vi "OCT Functinal Global.vi"(6 "Program Handle":T10, 7 "FFT States":T11, 8 "Error In":errorcluster, 9 "Input U16 Data":u16[][][](array[numeric]), 10 "Device In":T2, 11 "Dimension In":T4={"Depth"=1, "Height"=1000, "Width"=1024} {"Width" min=1; "Height" min=1; "Depth" min=1}) -> (0 "Error Out":errorcluster, 2 "Phase":sgl[][](array[numeric]), 3 "Magnitude":sgl[][](array[numeric]))   [LabVIEW 2012]
uses:
  User Controls/Array Dimensions.ctl
  Non-User VIs/Controls/Device ID.ctl
  OCT States.ctl
  Non-User VIs/Controls/Program Handle.ctl
  Non-User VIs/Controls/Memory Object.ctl
  Non-User VIs/Controls/Memory ID.ctl
  Non-User VIs/Controls/Memory Type.ctl
  Non-User VIs/FFT/FFT Control.ctl
  Non-User VIs/FFT/FFT Types.ctl
  Non-User VIs/FFT/FFT Dimension.ctl
  Non-User VIs/FFT/FFT Direction.ctl
  Non-User VIs/Allocate Memory/AllocateMemory_u16.vi
  Non-User VIs/Allocate Memory/AllocateMemory_32f.vi
  <vilib>/Analysis/4window.llb/Hanning Window (DBL).vi
  Non-User VIs/Write Memory/WriteMemory_32f.vi
  Non-User VIs/FFT/Create FFT Plan 32f.vi
  Non-User VIs/Write Memory/WriteMemory_u16.vi
  Non-User VIs/Set Kernel Arguments/Set Kernel Arguments Memory Object.vi
  Non-User VIs/Set Kernel Arguments/Set Kernel Arguments 32f.vi
  Non-User VIs/FFT/Compute FFT 32f.vi
  Non-User VIs/FFT/Delete FFT Plan 32f.vi
  Non-User VIs/Read Memory/ReadMemory_32f.vi
  OpenCLV x64.lvlib
  <vilib>/Analysis/NI_AALPro.lvlib
panel:
  out "Hanning Window":T1={"Device ID"=0, "Memeroy ID"=0, "Dimension"={"Depth"=1, "Height"=1, "Width"=1}, "Memory Type"=enum."32f"} {"Dimension"."Width" min=1; "Dimension"."Height" min=1; "Dimension"."Depth" min=1}
  out "FFT Object":T6 {"Imag"."Dimension"."Width" min=1; "Imag"."Dimension"."Height" min=1; "Imag"."Dimension"."Depth" min=1; "Real"."Dimension"."Width" min=1; "Real"."Dimension"."Height" min=1; "Real"."Dimension"."Depth" min=1}
  out "Program Handle 3":T10
  out "Pre FFT 32f":T1={"Device ID"=0, "Memeroy ID"=0, "Dimension"={"Depth"=1, "Height"=1, "Width"=1}, "Memory Type"=enum."32f"} {"Dimension"."Width" min=1; "Dimension"."Height" min=1; "Dimension"."Depth" min=1}
  out "u16 Input":T1={"Device ID"=0, "Memeroy ID"=0, "Dimension"={"Depth"=1, "Height"=1, "Width"=1}, "Memory Type"=enum."32f"} {"Dimension"."Width" min=1; "Dimension"."Height" min=1; "Dimension"."Depth" min=1}
  in  "Imag":T1={"Device ID"=0, "Memeroy ID"=0, "Dimension"={"Depth"=1, "Height"=1, "Width"=1}, "Memory Type"=enum."32f"} {"Dimension"."Width" min=1; "Dimension"."Height" min=1; "Dimension"."Depth" min=1}
  in  "Real":T1={"Device ID"=0, "Memeroy ID"=0, "Dimension"={"Depth"=1, "Height"=1, "Width"=1}, "Memory Type"=enum."32f"} {"Dimension"."Width" min=1; "Dimension"."Height" min=1; "Dimension"."Depth" min=1}
  out "Program Handle 2":T10
  # "Locals"
  # "Outputs"
  # "Inputs"
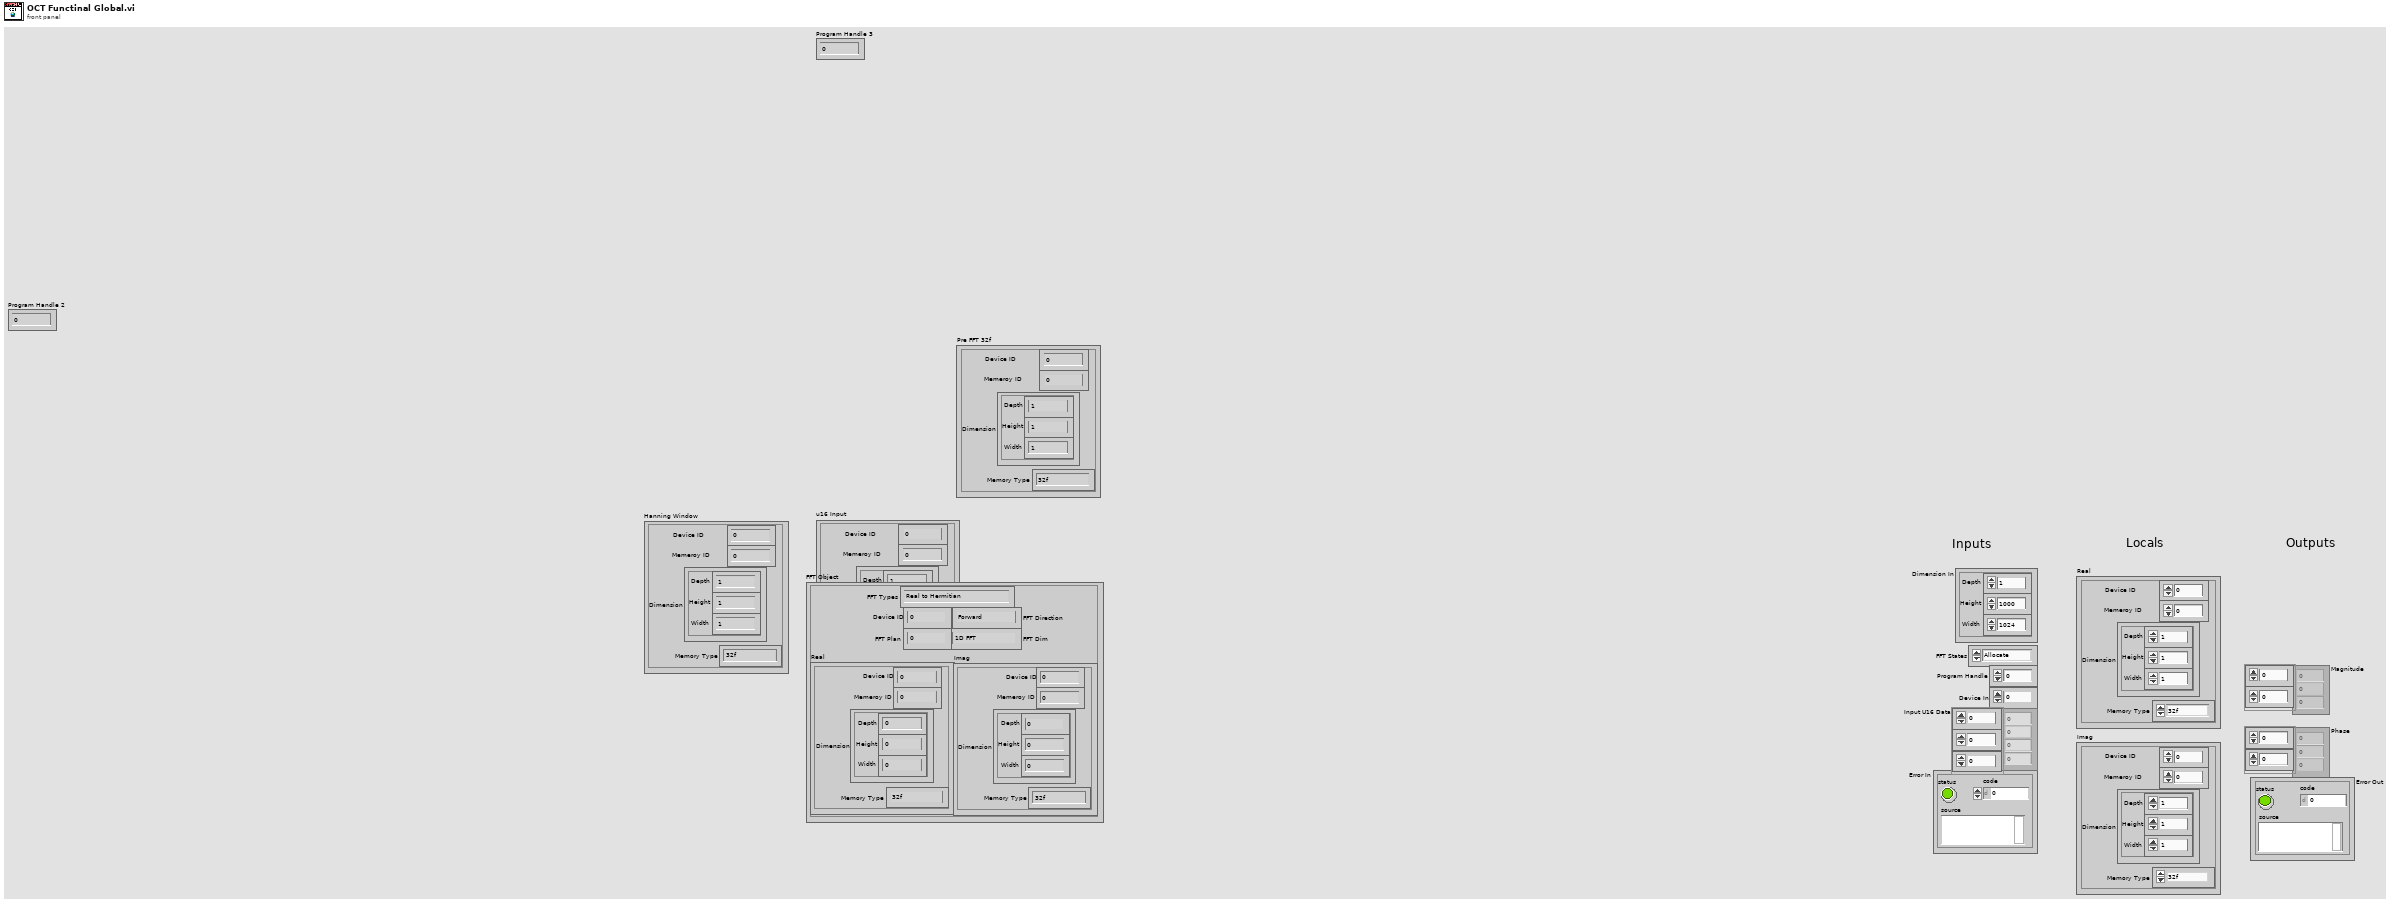
[diagram p1: front panel]
types:
  T1 = typedef "OpenCLV x64.lvlib/Memory Object.ctl" = cluster{"Device ID":T2, "Memeroy ID":T3, "Dimension":T4, "Memory Type":T5}
  T2 = typedef "OpenCLV x64.lvlib/Device ID.ctl" = u64
  T3 = typedef "OpenCLV x64.lvlib/Memory ID.ctl" = u64
  T4 = typedef "Array Dimensions.ctl" = cluster{"Depth":u64, "Height":u64, "Width":u64}
  T5 = typedef "OpenCLV x64.lvlib/Memory Type.ctl" = enum16{"32f", "u8", "i8", "u16", "i16", "u32", "i32", "64f"}
  T6 = typedef "OpenCLV x64.lvlib/FFT Control.ctl" = cluster{"Device ID":T2, "FFT Types":T7, "FFT Dim":T8, "Real":T1, "Imag":T1, "FFT Plan":u64, "FFT Direction":T9}
  T7 = typedef "OpenCLV x64.lvlib/FFT Types.ctl" = enum16{"Real to Hermitian", "Hermitian to Real", "Complex to Complex"}
  T8 = typedef "OpenCLV x64.lvlib/FFT Dimension.ctl" = enum16{"1D FFT", "2D FFT", "3D FFT"}
  T9 = typedef "OpenCLV x64.lvlib/FFT Direction.ctl" = enum16{"Forward", "Reverse"}
  T10 = typedef "OpenCLV x64.lvlib/Program Handle.ctl" = u64
  T11 = typedef "OCT States.ctl" = enum16{"Allocate", "Pre-FFT No Optimization", "Pre-FFT Global Memory", "Pre-FFT Local Memory", "FFT", "Post FFT", "Read Data", "Clean-up"}
  T12 = cluster{"Memory Object":T1, "Memory Object":T1, "Memory Object Out":T1, "FFT Object":T6, "Memory Object":T1, "Memory Object":T1, "Real":T1, "Imag":T1}
  T13 = typedef "OpenCLV x64.lvlib/Kernel Handle.ctl" = u64
  T14 = typedef "OpenCLV x64.lvlib/Kernel Workgroup Information.ctl" = cluster{"Compile Workgroup Size":u64[], "Kernel Private Mem":u64, "Kernel Local Mem":u64, "Work Group Multiple":u64, "Max Work Group Size":u64}
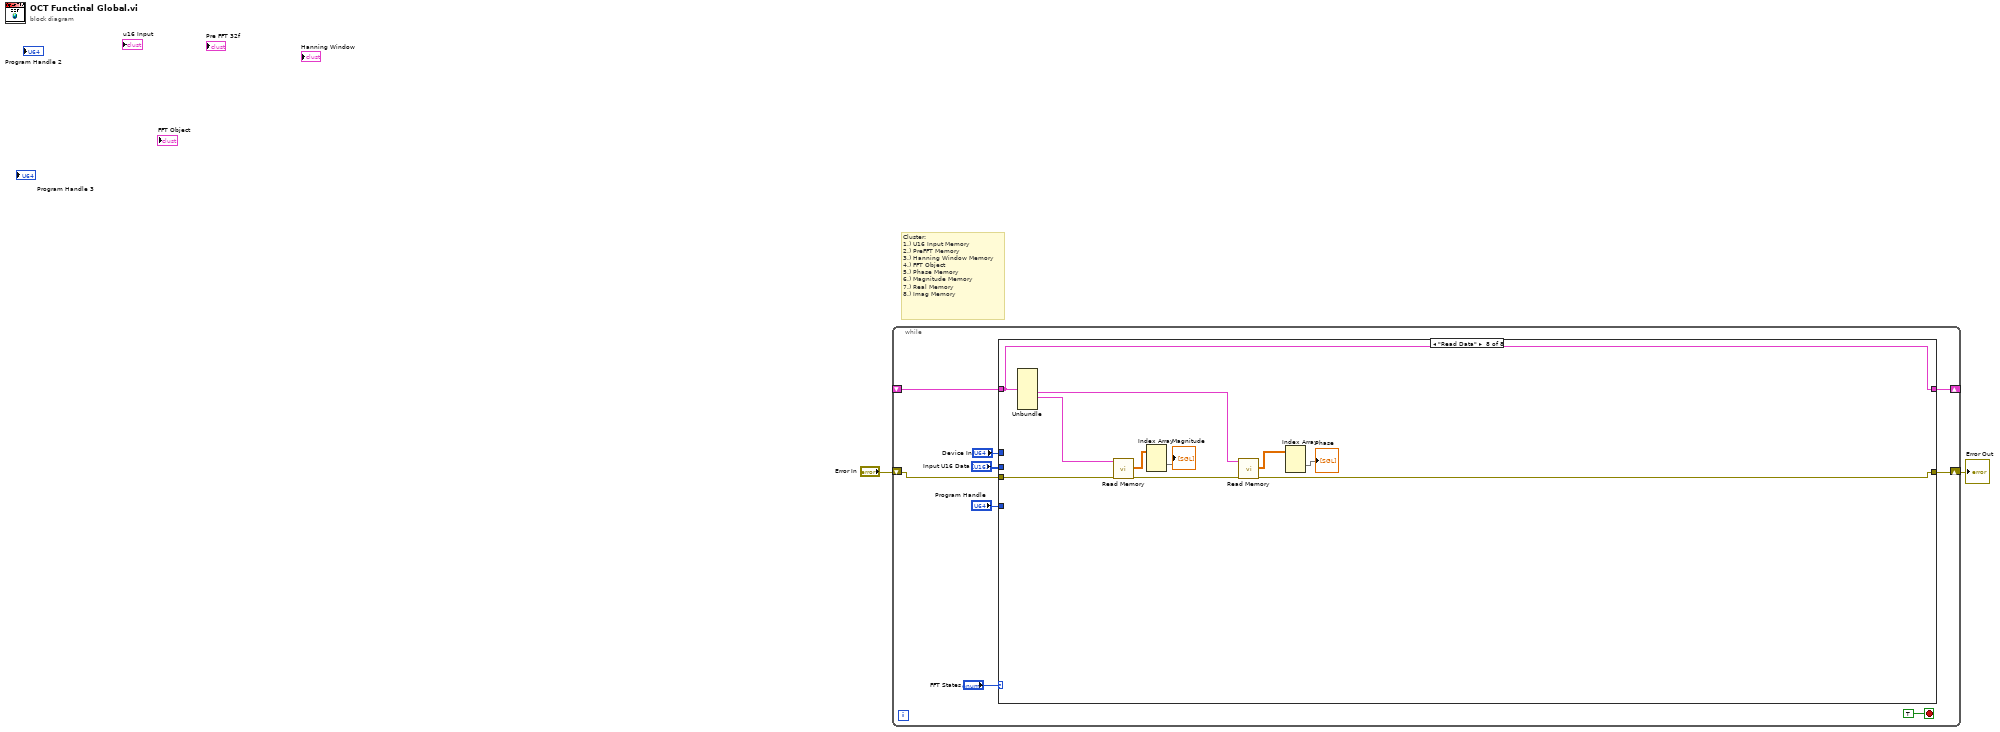
[diagram p0: block diagram]
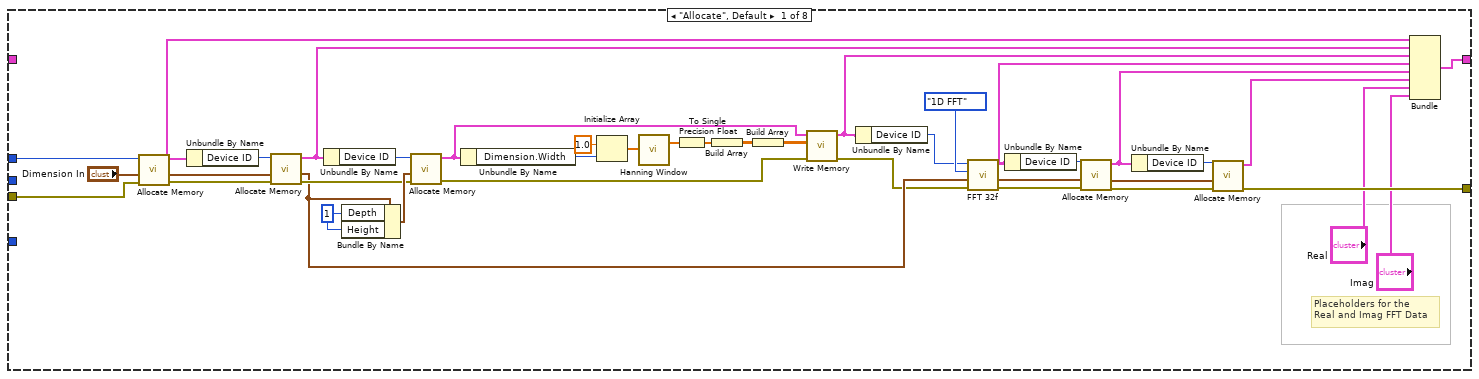
[diagram p2: hidden frame]
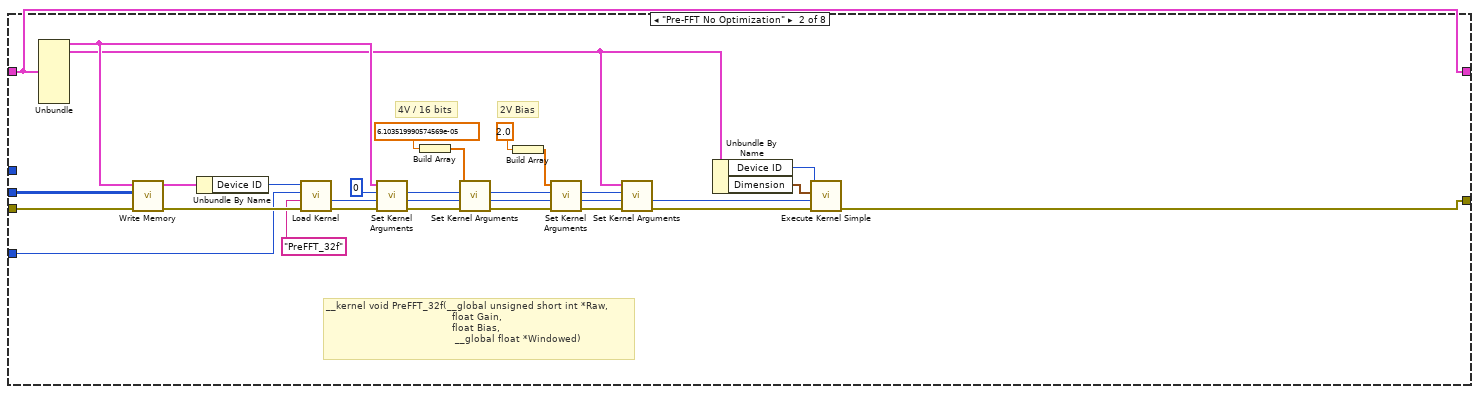
[diagram p3: hidden frame]
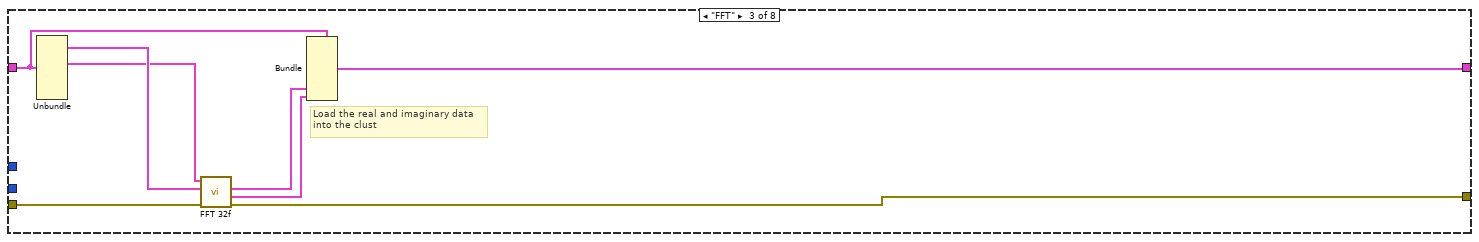
[diagram p4: hidden frame]
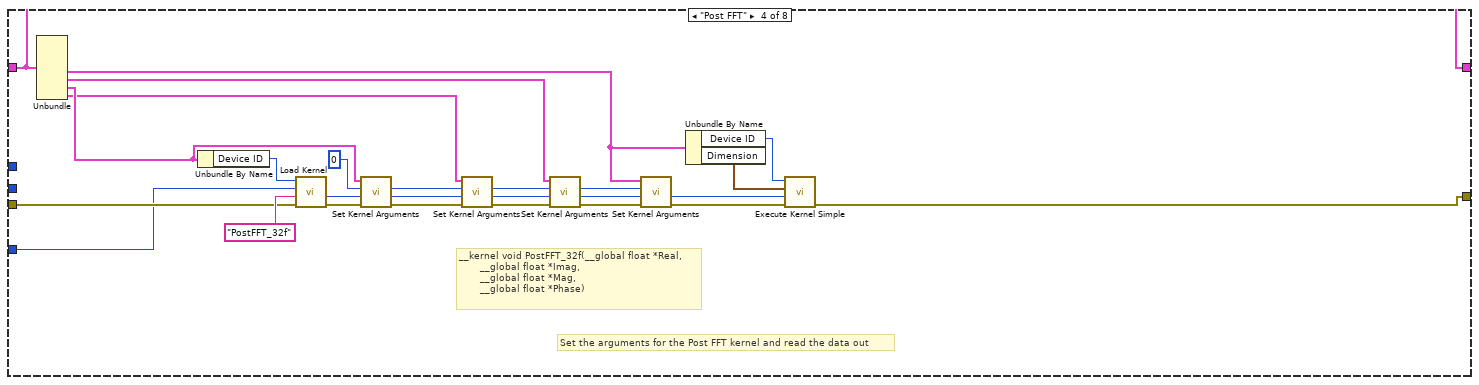
[diagram p5: hidden frame]
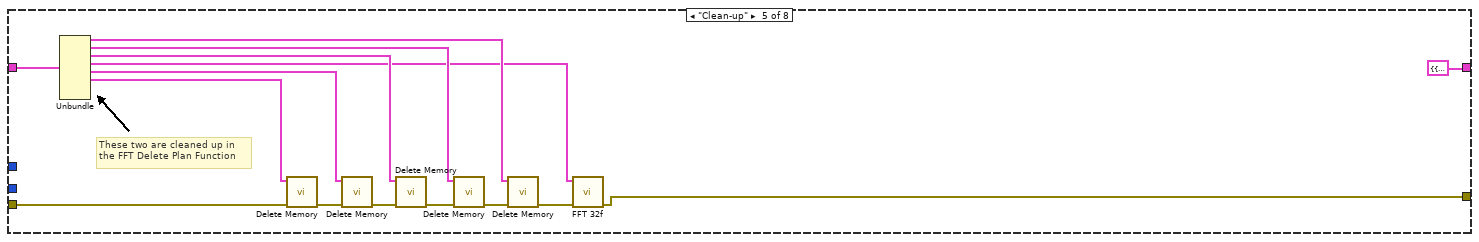
[diagram p6: hidden frame]
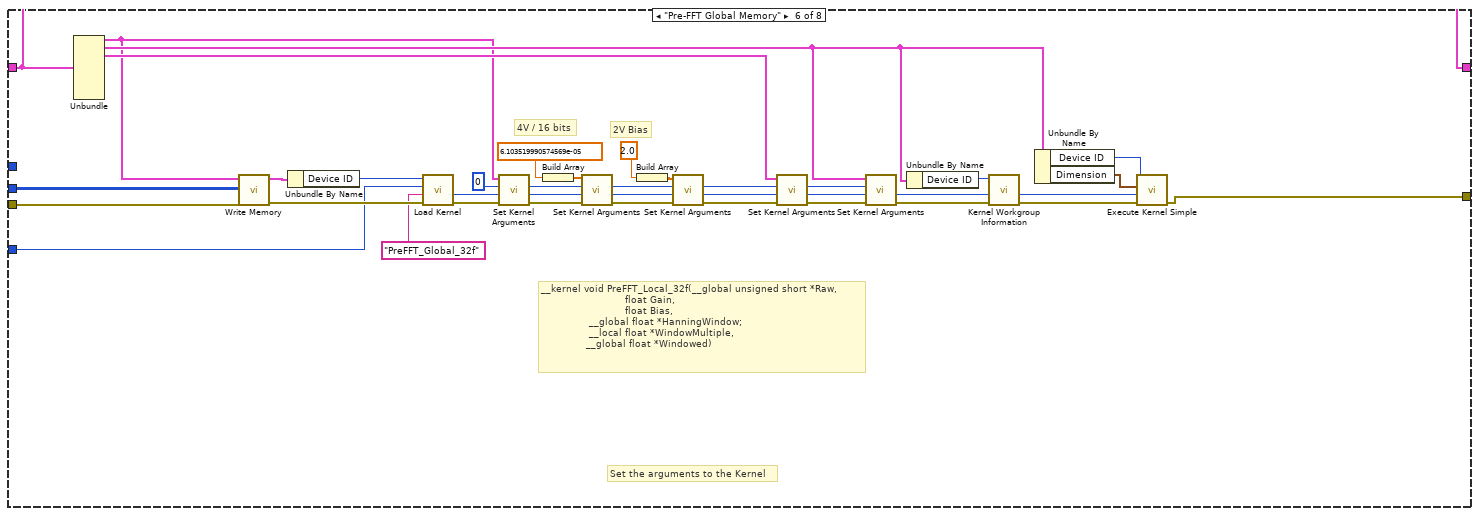
[diagram p7: hidden frame]
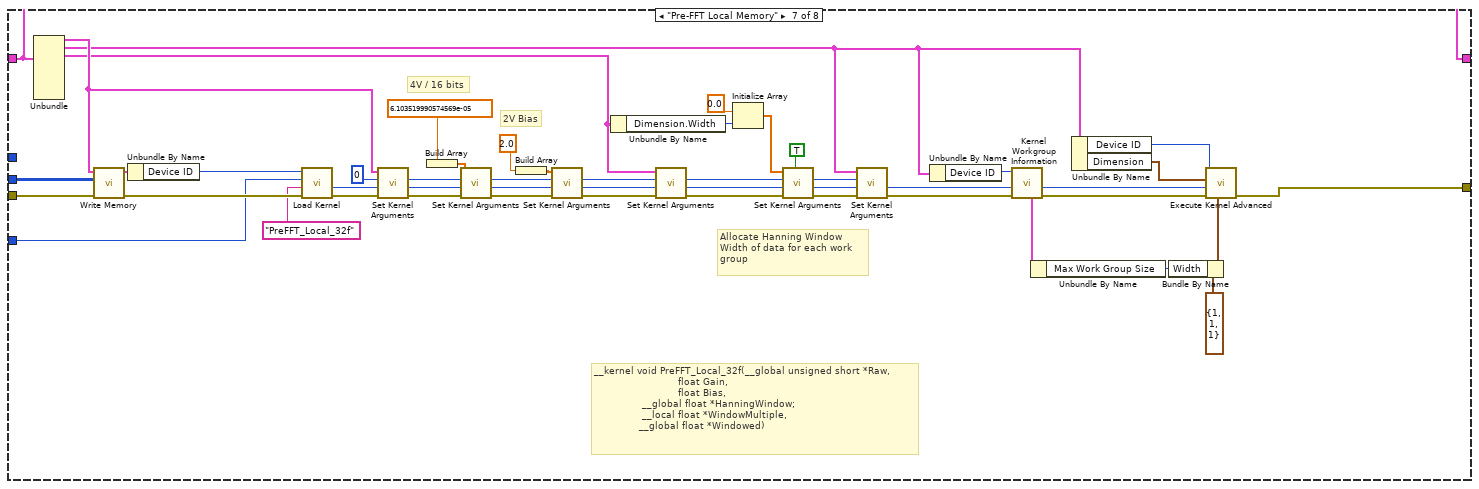
[diagram p8: hidden frame]
diagram:
  # "Cluster:\n1.) U16 Input Memory\n2.) PreFFT Memory\n3.) Hanning Window Memory\n4.) FFT Object\n5.) Phase Memory\n6.) Magnitude Memory\n7.) Real Memory\n8.) Imag Memory"
  n1 = while {
    shift-right: [w8] -> _
    shift-left: _ -> [w7]
    shift-right: [w6] -> w1
    shift-left: "Error In" -> [w5]
    stop <- TRUE stop-if-true
    n2 = case shown="\"Read Data\"" "FFT States" {
      tunnel: "Device In" -> [w27 _ _ _ _ _ _ _]
      tunnel: [w16 w56 w82 w92 T12 {"Memory Object"={"Device ID"=0, "Memeroy ID"=0, "Dimension"={"Depth"=0, "Height"=0, "Width"=0}, "Memory Type"=enum."32f"}, "Memory Object"={"Device ID"=0, "Memeroy ID"=0, "Dimension"={"Depth"=0, "Height"=0, "Width"=0}, "Memory Type"=enum."32f"}, "Memory Object Out"={"Device ID"=0, "Memeroy ID"=0, "Dimension"={"Depth"=0, "Height"=0, "Width"=0}, "Memory Type"=enum."32f"}, "FFT Object"={"Device ID"=0, "FFT Types"=enum."Real to Hermitian", "FFT Dim"=enum."1D FFT", "Real"={"Device ID"=0, "Memeroy ID"=0, "Dimension"={"Depth"=0, "Height"=0, "Width"=0}, "Memory Type"=enum."32f"}, "Imag"={"Device ID"=0, "Memeroy ID"=0, "Dimension"={"Depth"=0, "Height"=0, "Width"=0}, "Memory Type"=enum."32f"}, "FFT Plan"=0, "FFT Direction"=enum."Forward"}, "Memory Object"={"Device ID"=0, "Memeroy ID"=0, "Dimension"={"Depth"=0, "Height"=0, "Width"=0}, "Memory Type"=enum."32f"}, "Memory Object"={"Device ID"=0, "Memeroy ID"=0, "Dimension"={"Depth"=0, "Height"=0, "Width"=0}, "Memory Type"=enum."32f"}, "Real"={"Device ID"=0, "Memeroy ID"=0, "Dimension"={"Depth"=0, "Height"=0, "Width"=0}, "Memory Type"=enum."32f"}, "Imag"={"Device ID"=0, "Memeroy ID"=0, "Dimension"={"Depth"=0, "Height"=0, "Width"=0}, "Memory Type"=enum."32f"}} ("Cluster") w133 w217 w218] -> w8
      tunnel: w7 -> [_ w56 w85 w92 w129 w133 w217 w218]
      tunnel: w5 -> [w15 w58 w89 w97 w116 w139 w177 w225]
      tunnel: [w14 w55 w86 w91 w117 w134 w171 w222] -> w6
      tunnel: "Program Handle" -> [_ w57 _ w90 _ w135 w175 _]
      tunnel: "Input U16 Data" -> [_ w52 _ _ _ w131 w176 _]
      frame "Allocate", Default {
        w42 = u64 1 ("Depth")
        # "Placeholders for the \nReal and Imag FFT Data"
        n3 = call-poly "Allocate Memory.vi"("Error In"=w15, "Dimension"="Dimension In", "Device In"=w27) -> ("Error Out"=w35:errorcluster, "Dimension Out"=w36:T4, "Memory Object"=w24:T1)  [unwired: 6 in]
        n4 = Unbundle By Name(w24) -> ("Device ID"=w34:T2)
        n5 = call-poly "Allocate Memory.vi"("Error In"=w35, "Dimension"=w36, "Device In"=w34) -> ("Error Out"=w39:errorcluster, "Dimension Out"=w23:T4, "Memory Object"=w26:T1)  [unwired: 6 in]
        n6 = Unbundle By Name(w26) -> ("Device ID"=w43:T2)
        n7 = Bundle By Name(cluster=w23, "Depth"=w42, "Height"=w42) -> (w40:T4)
        n8 = call-poly "Allocate Memory.vi"("Error In"=w39, "Dimension"=w40, "Device In"=w43) -> ("Error Out"=w28:errorcluster, "Memory Object"=w25:T1)  [unwired: 6 in, 1 out]
        n9 = Unbundle By Name(w25) -> ("Dimension.Width"=w48:u64)
        n10 = Initialize Array(1.0 ("element"), w48) -> (w49:dbl[])
        n11 = call-poly <vilib>:"Hanning Window.vi"("X"=w49) -> ("Windowed X"=w46:dbl[])  [unwired: 1 out]
        n12 = To Single Precision Float(number=w46) -> (single precision float=w45:sgl[])
        n13 = Build Array(w45) -> (w44:sgl[][])
        n14 = Build Array(w44) -> (w50:sgl[][][])
        n15 = call-poly "Write Memory.vi"("Error In"=w28, "Data In"=w50, "Memory Object In"=w25) -> ("Error Out"=w22:errorcluster, "Memory Object Out"=w21:T1)  [unwired: 6 in, 1 out]
        n16 = Unbundle By Name(w21) -> ("Device ID"=w20:T2)
        n17 = call-poly "FFT 32f.vi"("Error In"=w22, "Dimension"=w23, "FFT Dimension"=FFT_Dimension."1D FFT", "Labview Device"=w20) -> ("Error Out"=w30:errorcluster, "FFT Output Dimensions"=w37:T4, "FFT Object"=w19:T6)  [unwired: 5 in]
        n18 = Unbundle By Name(w19) -> ("Device ID"=w38:T2)
        n19 = call-poly "Allocate Memory.vi"("Error In"=w30, "Dimension"=w37, "Device In"=w38) -> ("Error Out"=w33:errorcluster, "Dimension Out"=w32:T4, "Memory Object"=w18:T1)  [unwired: 6 in]
        n20 = Unbundle By Name(w18) -> ("Device ID"=w31:T2)
        n21 = call-poly "Allocate Memory.vi"("Error In"=w33, "Dimension"=w32, "Device In"=w31) -> ("Error Out"=w14:errorcluster, "Memory Object"=w17:T1)  [unwired: 6 in, 1 out]
        n22 = Bundle("Memory Object"=w24, "Memory Object"=w26, "Memory Object Out"=w21, "FFT Object"=w19, "Memory Object"=w18, "Memory Object"=w17, "Real"="Real", "Imag"="Imag") -> (w16:T12)  [unwired: 1 in]
      }
      frame "Pre-FFT No Optimization" {
        # "2V Bias"
        # "4V / 16 bits"
        # "__kernel void PreFFT_32f(__global unsigned short int *Raw,\n                                          float Gain,\n                                          float Bias,\n\t\t\t                                        __global float *Windowed)"
        n23 = Unbundle(w56) -> ("Memory Object"=w53:T1, "Memory Object"=w51:T1)  [unwired: 6 out]
        n24 = call-poly "Write Memory.vi"("Error In"=w58, "Data In"=w52, "Memory Object In"=w53) -> ("Error Out"=w69:errorcluster, "Memory Object Out"=w54:T1)  [unwired: 7 in]
        n25 = Unbundle By Name(w54) -> ("Device ID"=w78:T2)
        n26 = call "Load Kernel.vi"("Error In"=w69, "Kernel Name"="PreFFT_32f", "Program Handle"=w57, "Device In"=w78) -> ("Error Out"=w81:errorcluster, "Kernel Handle"=w80:T13)  [unwired: 4 in, 2 out]
        n27 = call-poly "Set Kernel Arguments.vi"("Error In"=w81, "Kernel Handle"=w80, "Argument Number"=0, "Memory Object"=w53) -> ("Error Out"=w60:errorcluster, "Kernel Handle out"=w72:T13, "Auto Inc Arugment Number"=w73:i32)  [unwired: 5 in]
        n28 = Build Array(sgl 6.10352e-05 ("x")) -> (w61:sgl[])
        n29 = call-poly "Set Kernel Arguments.vi"("Error In"=w60, "Kernel Handle"=w72, "Argument Number"=w73, "32f Constant"=w61) -> ("Error Out"=w63:errorcluster, "Kernel Handle out"=w71:T13, "Auto Inc Arugment Number"=w74:i32)  [unwired: 5 in]
        n30 = Build Array(sgl 2.0 ("x")) -> (w62:sgl[])
        n31 = call-poly "Set Kernel Arguments.vi"("Error In"=w63, "Kernel Handle"=w71, "Argument Number"=w74, "32f Constant"=w62) -> ("Error Out"=w64:errorcluster, "Kernel Handle out"=w65:T13, "Auto Inc Arugment Number"=w66:i32)  [unwired: 5 in]
        n32 = call-poly "Set Kernel Arguments.vi"("Error In"=w64, "Kernel Handle"=w65, "Argument Number"=w66, "Memory Object"=w51) -> ("Error Out"=w67:errorcluster, "Kernel Handle out"=w77:T13)  [unwired: 5 in, 1 out]
        n33 = Unbundle By Name(w51) -> ("Device ID"=w68:T2, "Dimension"=w70:T4)
        n34 = call "Execute Kernel Simple.vi"("Error In"=w67, "Kernel Handle"=w77, "Thread Dimensions"=w70, "Device In"=w68) -> ("Error Out"=w55:errorcluster)  [unwired: 4 in, 3 out]
      }
      frame "FFT" {
        # "Load the real and imaginary data\ninto the clust"
        n35 = Unbundle(w85) -> ("Memory Object"=w88:T1, "FFT Object"=w87:T6)  [unwired: 6 out]
        n36 = call-poly "FFT 32f.vi"("Error In"=w89, "Real In"=w88, "FFT Object"=w87) -> ("Error Out"=w86:errorcluster, "Imag Out"=w84:T1, "Real Out"=w83:T1)  [unwired: 4 in, 2 out]
        n37 = Bundle(cluster=w85, "Real"=w83, "Imag"=w84) -> (w82:T12)  [unwired: 6 in]
      }
      frame "Post FFT" {
        # "Set the arguments for the Post FFT kernel and read the data out"
        # "__kernel void PostFFT_32f(__global float *Real,\n\t\t\t    __global float *Imag,\n\t\t\t    __global float *Mag,\n    \t\t\t__global float *Phase)"
        n38 = Unbundle(w92) -> ("Memory Object"=w93:T1, "Memory Object"=w94:T1, "Real"=w96:T1, "Imag"=w95:T1)  [unwired: 4 out]
        n39 = Unbundle By Name(w96) -> ("Device ID"=w115:T2)
        n40 = call "Load Kernel.vi"("Error In"=w97, "Kernel Name"="PostFFT_32f", "Program Handle"=w90, "Device In"=w115) -> ("Error Out"=w99:errorcluster, "Kernel Handle"=w112:T13)  [unwired: 4 in, 2 out]
        n41 = call-poly "Set Kernel Arguments.vi"("Error In"=w99, "Kernel Handle"=w112, "Argument Number"=0, "Memory Object"=w96) -> ("Error Out"=w102:errorcluster, "Kernel Handle out"=w101:T13, "Auto Inc Arugment Number"=w100:i32)  [unwired: 5 in]
        n42 = call-poly "Set Kernel Arguments.vi"("Error In"=w102, "Kernel Handle"=w101, "Argument Number"=w100, "Memory Object"=w95) -> ("Error Out"=w103:errorcluster, "Kernel Handle out"=w104:T13, "Auto Inc Arugment Number"=w105:i32)  [unwired: 5 in]
        n43 = call-poly "Set Kernel Arguments.vi"("Error In"=w103, "Kernel Handle"=w104, "Argument Number"=w105, "Memory Object"=w94) -> ("Error Out"=w106:errorcluster, "Kernel Handle out"=w107:T13, "Auto Inc Arugment Number"=w108:i32)  [unwired: 5 in]
        n44 = call-poly "Set Kernel Arguments.vi"("Error In"=w106, "Kernel Handle"=w107, "Argument Number"=w108, "Memory Object"=w93) -> ("Error Out"=w109:errorcluster, "Kernel Handle out"=w114:T13)  [unwired: 5 in, 1 out]
        n45 = Unbundle By Name(w93) -> ("Device ID"=w110:T2, "Dimension"=w113:T4)
        n46 = call "Execute Kernel Simple.vi"("Error In"=w109, "Kernel Handle"=w114, "Thread Dimensions"=w113, "Device In"=w110) -> ("Error Out"=w91:errorcluster)  [unwired: 4 in, 3 out]
      }
      frame "Clean-up" {
        # "These two are cleaned up in\nthe FFT Delete Plan Function"
        n47 = Unbundle(w129) -> ("Memory Object"=w120:T1, "Memory Object"=w122:T1, "Memory Object Out"=w124:T1, "FFT Object"=w118:T6, "Memory Object"=w126:T1, "Memory Object"=w128:T1)  [unwired: 2 out]
        n48 = call "Delete Memory.vi"("Error In"=w116, "Memory Object In"=w128) -> ("Error Out"=w127:errorcluster)  [unwired: 8 in, 1 out]
        n49 = call "Delete Memory.vi"("Error In"=w127, "Memory Object In"=w126) -> ("Error Out"=w125:errorcluster)  [unwired: 8 in, 1 out]
        n50 = call "Delete Memory.vi"("Error In"=w125, "Memory Object In"=w124) -> ("Error Out"=w123:errorcluster)  [unwired: 8 in, 1 out]
        n51 = call "Delete Memory.vi"("Error In"=w123, "Memory Object In"=w122) -> ("Error Out"=w121:errorcluster)  [unwired: 8 in, 1 out]
        n52 = call "Delete Memory.vi"("Error In"=w121, "Memory Object In"=w120) -> ("Error Out"=w119:errorcluster)  [unwired: 8 in, 1 out]
        n53 = call-poly "FFT 32f.vi"("Error In"=w119, "FFT Object"=w118) -> ("Error Out"=w117:errorcluster)  [unwired: 9 in]
      }
      frame "Pre-FFT Global Memory" {
        # "2V Bias"
        # "4V / 16 bits"
        # "Set the arguments to the Kernel"
        # "__kernel void PreFFT_Local_32f(__global unsigned short *Raw,\n                           \tfloat Gain,\n                           \tfloat Bias,\n\t\t\t\t\t\t\t         __global float *HanningWindow;\n\t\t\t\t            __local float *WindowMultiple,\n\t\t           \t __global float *Windowed)"
        n54 = Unbundle(w133) -> ("Memory Object"=w132:T1, "Memory Object"=w137:T1, "Memory Object Out"=w138:T1)  [unwired: 5 out]
        n55 = call-poly "Write Memory.vi"("Error In"=w139, "Data In"=w131, "Memory Object In"=w132) -> ("Error Out"=w164:errorcluster, "Memory Object Out"=w136:T1)  [unwired: 7 in]
        n56 = Unbundle By Name(w136) -> ("Device ID"=w152:T2)
        n57 = call "Load Kernel.vi"("Error In"=w164, "Kernel Name"="PreFFT_Global_32f", "Program Handle"=w135, "Device In"=w152) -> ("Error Out"=w155:errorcluster, "Kernel Handle"=w154:T13)  [unwired: 4 in, 2 out]
        n58 = call-poly "Set Kernel Arguments.vi"("Error In"=w155, "Kernel Handle"=w154, "Argument Number"=0, "Memory Object"=w132) -> ("Error Out"=w141:errorcluster, "Kernel Handle out"=w147:T13, "Auto Inc Arugment Number"=w148:i32)  [unwired: 5 in]
        n59 = Build Array(sgl 6.10352e-05 ("x")) -> (w142:sgl[])
        n60 = call-poly "Set Kernel Arguments.vi"("Error In"=w141, "Kernel Handle"=w147, "Argument Number"=w148, "32f Constant"=w142) -> ("Error Out"=w144:errorcluster, "Kernel Handle out"=w146:T13, "Auto Inc Arugment Number"=w149:i32)  [unwired: 5 in]
        n61 = Build Array(sgl 2.0 ("x")) -> (w143:sgl[])
        n62 = call-poly "Set Kernel Arguments.vi"("Error In"=w144, "Kernel Handle"=w146, "Argument Number"=w149, "32f Constant"=w143) -> ("Error Out"=w161:errorcluster, "Kernel Handle out"=w162:T13, "Auto Inc Arugment Number"=w163:i32)  [unwired: 5 in]
        n63 = call-poly "Set Kernel Arguments.vi"("Error In"=w161, "Kernel Handle"=w162, "Argument Number"=w163, "Memory Object"=w138) -> ("Error Out"=w166:errorcluster, "Kernel Handle out"=w167:T13, "Auto Inc Arugment Number"=w168:i32)  [unwired: 5 in]
        n64 = call-poly "Set Kernel Arguments.vi"("Error In"=w166, "Kernel Handle"=w167, "Argument Number"=w168, "Memory Object"=w137) -> ("Error Out"=w156:errorcluster, "Kernel Handle out"=w157:T13)  [unwired: 5 in, 1 out]
        n65 = Unbundle By Name(w137) -> ("Device ID"=w160:T2)
        n66 = call "Kernel Workgroup Information.vi"("Error In"=w156, "Kernel Handle"=w157, "Device ID"=w160) -> ("Error Out"=w158:errorcluster, "Kernel Handle"=w159:T13)  [unwired: 5 in, 2 out]
        n67 = Unbundle By Name(w137) -> ("Device ID"=w145:T2, "Dimension"=w165:T4)
        n68 = call "Execute Kernel Simple.vi"("Error In"=w158, "Kernel Handle"=w159, "Thread Dimensions"=w165, "Device In"=w145) -> ("Error Out"=w134:errorcluster)  [unwired: 4 in, 3 out]
      }
      frame "Pre-FFT Local Memory" {
        # "Allocate Hanning Window\nWidth of data for each work\ngroup"
        # "2V Bias"
        # "4V / 16 bits"
        # "__kernel void PreFFT_Local_32f(__global unsigned short *Raw,\n                           \tfloat Gain,\n                           \tfloat Bias,\n\t\t\t\t\t\t\t         __global float *HanningWindow;\n\t\t\t\t            __local float *WindowMultiple,\n\t\t           \t __global float *Windowed)"
        n69 = Unbundle(w217) -> ("Memory Object"=w173:T1, "Memory Object"=w172:T1, "Memory Object Out"=w170:T1)  [unwired: 5 out]
        n70 = call-poly "Write Memory.vi"("Error In"=w177, "Data In"=w176, "Memory Object In"=w173) -> ("Error Out"=w190:errorcluster, "Memory Object Out"=w174:T1)  [unwired: 7 in]
        n71 = Unbundle By Name(w174) -> ("Device ID"=w180:T2)
        n72 = call "Load Kernel.vi"("Error In"=w190, "Kernel Name"="PreFFT_Local_32f", "Program Handle"=w175, "Device In"=w180) -> ("Error Out"=w182:errorcluster, "Kernel Handle"=w181:T13)  [unwired: 4 in, 2 out]
        n73 = call-poly "Set Kernel Arguments.vi"("Error In"=w182, "Kernel Handle"=w181, "Argument Number"=0, "Memory Object"=w173) -> ("Error Out"=w194:errorcluster, "Kernel Handle out"=w199:T13, "Auto Inc Arugment Number"=w200:i32)  [unwired: 5 in]
        n74 = Build Array(sgl 6.10352e-05 ("x")) -> (w195:sgl[])
        n75 = call-poly "Set Kernel Arguments.vi"("Error In"=w194, "Kernel Handle"=w199, "Argument Number"=w200, "32f Constant"=w195) -> ("Error Out"=w197:errorcluster, "Kernel Handle out"=w198:T13, "Auto Inc Arugment Number"=w201:i32)  [unwired: 5 in]
        n76 = Build Array(sgl 2.0 ("x")) -> (w196:sgl[])
        n77 = call-poly "Set Kernel Arguments.vi"("Error In"=w197, "Kernel Handle"=w198, "Argument Number"=w201, "32f Constant"=w196) -> ("Error Out"=w209:errorcluster, "Kernel Handle out"=w210:T13, "Auto Inc Arugment Number"=w211:i32)  [unwired: 5 in]
        n78 = Unbundle By Name(w170) -> ("Dimension.Width"=w169:u64)
        n79 = call-poly "Set Kernel Arguments.vi"("Error In"=w209, "Kernel Handle"=w210, "Argument Number"=w211, "Memory Object"=w170) -> ("Error Out"=w212:errorcluster, "Kernel Handle out"=w213:T13, "Auto Inc Arugment Number"=w214:i32)  [unwired: 5 in]
        n80 = Initialize Array(sgl 0.0 ("element"), w169) -> (w216:sgl[])
        n81 = call-poly "Set Kernel Arguments.vi"("Local Data?"=TRUE, "Error In"=w212, "Kernel Handle"=w213, "Argument Number"=w214, "32f Constant"=w216) -> ("Error Out"=w206:errorcluster, "Kernel Handle out"=w207:T13, "Auto Inc Arugment Number"=w208:i32)  [unwired: 4 in]
        n82 = call-poly "Set Kernel Arguments.vi"("Error In"=w206, "Kernel Handle"=w207, "Argument Number"=w208, "Memory Object"=w172) -> ("Error Out"=w183:errorcluster, "Kernel Handle out"=w184:T13)  [unwired: 5 in, 1 out]
        n83 = Unbundle By Name(w172) -> ("Device ID"=w187:T2)
        n84 = call "Kernel Workgroup Information.vi"("Error In"=w183, "Kernel Handle"=w184, "Device ID"=w187) -> ("Error Out"=w185:errorcluster, "Kernel Handle"=w186:T13, "Kernel Information"=w191:T14)  [unwired: 5 in, 1 out]
        n85 = Unbundle By Name(w191) -> ("Max Work Group Size"=w193:u64)
        n86 = Unbundle By Name(w172) -> ("Device ID"=w179:T2, "Dimension"=w192:T4)
        n87 = Bundle By Name(cluster=T4 {"Depth"=1, "Height"=1, "Width"=1} ("Local Work Size"), "Width"=w193) -> (w188:T4)
        n88 = call "Execute Kernel Advanced.vi"("Local Work Size"=w188, "Error In"=w185, "Kernel Handle"=w186, "Thread Dimensions"=w192, "Device In"=w179) -> ("Error Out"=w171:errorcluster)  [unwired: 3 in, 3 out]
      }
      frame "Read Data" {
        n89 = Unbundle(w218) -> ("Memory Object"=w219:T1, "Memory Object"=w220:T1)  [unwired: 6 out]
        n90 = call-poly "Read Memory.vi"("Error In"=w225, "Memory Object In"=w220) -> ("Error Out"=w226:errorcluster, "Data Out"=w227:sgl[][][])  [unwired: 6 in, 2 out]
        n91 = Index Array(array=w227) -> (element=→"Magnitude":sgl[][])  [unwired: 3 in]
        n92 = call-poly "Read Memory.vi"("Error In"=w226, "Memory Object In"=w219) -> ("Error Out"=w222:errorcluster, "Data Out"=w223:sgl[][][])  [unwired: 6 in, 2 out]
        n93 = Index Array(array=w223) -> (element=→"Phase":sgl[][])  [unwired: 3 in]
      }
    }
  }
  "Error Out" <- w1
